vi "Write Pulse Driver Configuration.vi"(8 "error in (no error)":errorcluster, 10 "Pulse Driver Configuration":T1={"Post-trigger delay"=0.01, "Post-trigger duration"=0.1, "Rate"=1000000.0, "Ranges"=[10.0], "Re-name channels"=[], "Active channels"="0:1", "External clock"=FALSE} {"Rate" format="%#_8pHz"; "Post-trigger duration" format="%#_6ps"; "Post-trigger delay" format="%#_6ps"; "Ranges" format="%#_6pV"}, 11 "Micron Optics Driver in":refnum<class "Micron Optics Driver.lvclass">) -> (0 "error out":errorcluster, 3 "Micron Optics Driver out":refnum<class "Micron Optics Driver.lvclass">)   [LabVIEW 2024, in "Micron Optics Driver.lvclass"]
uses:
  Micron Optics Driver.lvclass
  Micron Optics Driver.lvclass/Micron Optics Driver.ctl
  Pulse Driver/Pusle Driver Configuration.ctl
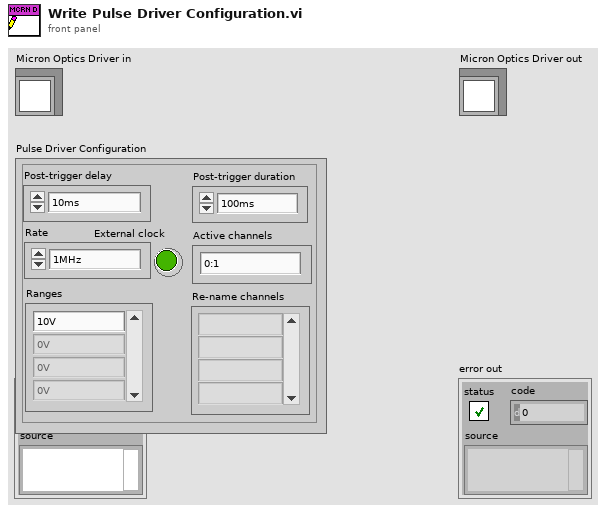
[diagram p1: front panel]
types:
  T1 = typedef "Pusle Driver Configuration.ctl" = cluster{"Post-trigger delay":dbl, "Post-trigger duration":dbl, "Rate":dbl, "Ranges":dbl[], "Re-name channels":string[], "Active channels":string, "External clock":bool}
  T2 = typedef "Micron optics didgitizer configuration.ctl" = cluster{"Post-trigger delay":dbl, "Post-trigger duration":dbl, "Rate":dbl, "Ranges":dbl[], "Re-name channels":string[], "Active channels":string, "External\nclock":bool, "Reference channel":i32, "Detection Setting IDs":u8[], "Stream and average":bool, "Address":string, "Number of sensors":i32}
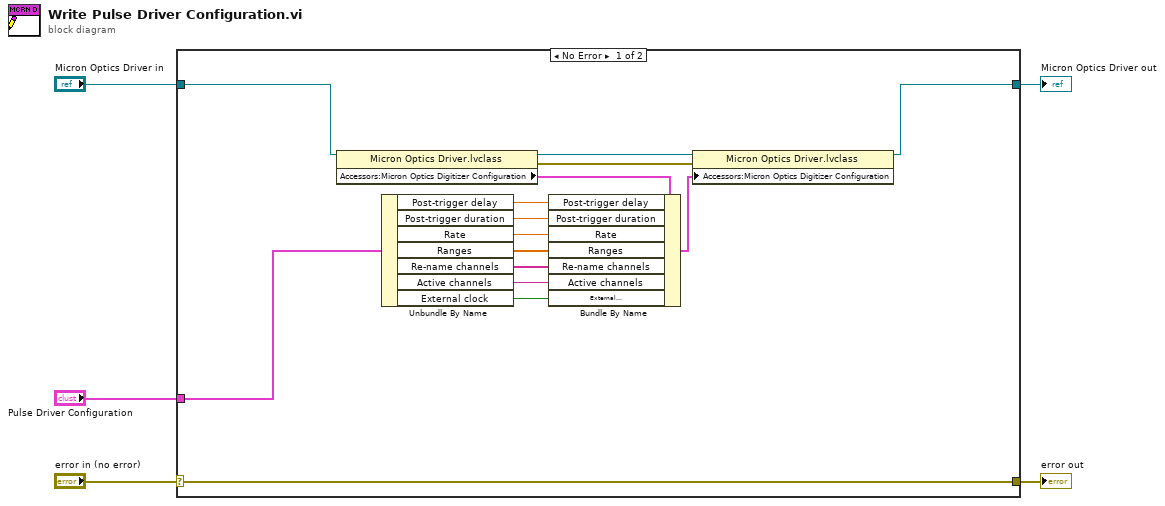
[diagram p0: block diagram]
diagram:
  n1 = case shown="No Error" "error in (no error)" {
    selector: "error in (no error)" -> [w20 w21]
    tunnel: [w20 w21] -> w4
    tunnel: [w11 w22] -> w2
    tunnel: "Micron Optics Driver in" -> [w10 w22]
    tunnel: "Pulse Driver Configuration" -> [w9 _]
    frame No Error {
      n2 = property class="Micron Optics Driver.lvclass"(reference=w10) -> (reference out=w12:refnum<class "Micron Optics Driver.lvclass">, error out=w19:errorcluster, "Accessors:Micron Optics Digitizer Configuration"=w13:T2)  [unwired: 1 in]
      n3 = Unbundle By Name(w9) -> ("Post-trigger delay"=w18:dbl, "Post-trigger duration"=w17:dbl, "Rate"=w16:dbl, "Ranges"=w15:dbl[], "Re-name channels"=w6:string[], "Active channels"=w7:string, "External clock"=w8:bool)
      n4 = Bundle By Name(cluster=w13, "Post-trigger delay"=w18, "Post-trigger duration"=w17, "Rate"=w16, "Ranges"=w15, "Re-name channels"=w6, "Active channels"=w7, "External\nclock"=w8) -> (w14:T2)
      n5 = property class="Micron Optics Driver.lvclass"(reference=w12, error in=w19, "Accessors:Micron Optics Digitizer Configuration"=w14) -> (reference out=w11:refnum<class "Micron Optics Driver.lvclass">)  [unwired: 1 out]
    }
    frame Error {
    }
  }
  "error out" <- w4
  "Micron Optics Driver out" <- w2
